vi "Actor Core.vi"(8 "error in":errorcluster, 11 "Menu View in":refnum<class "Menu View.lvclass">) -> (0 "error out":errorcluster, 3 "Actor out":refnum<class "Actor.lvclass">)   [LabVIEW 2020, in "Menu View.lvlib" / "Menu View.lvclass"]
doc: "(<B>Filename</B>: Actor Framework.lvlib:Actor.lvclass:Actor Core.vi)\n\nReceives messages to the actor, reacts to them, and initiates any error handling that may shut the actor down.\n\nDescendant classes may override this VI to append parallel tasks for the actor to complete while it handles messages. Overrides use the Call Parent Method node."
uses:
  Menu View.lvclass
  C:/Program Files/National Instruments/LabVIEW 2020/vi.lib/ActorFramework/Actor/Actor.lvclass
  <vilib>/ActorFramework/Actor/Actor.lvclass
  Menu View.lvclass/Menu View.ctl
  <vilib>/ActorFramework/Actor/Actor.lvclass/Actor.ctl
  <vilib>/ActorFramework/Message Enqueuer/Message Enqueuer.lvclass/Message Enqueuer.ctl
  Menu View Messages/Broadcast Menu Pressed Msg/Broadcast Menu Pressed Msg.lvclass/Broadcast Menu Pressed Msg.ctl
  Menu View Messages/Broadcast Tools Pressed Msg/Broadcast Tools Pressed Msg.lvclass/Broadcast Tools Pressed Msg.ctl
  Menu View Messages/Broadcast Help Pressed Msg/Broadcast Help Pressed Msg.lvclass/Broadcast Help Pressed Msg.ctl
  Menu View Messages/Broadcast Undo Pressed Msg/Broadcast Undo Pressed Msg.lvclass/Broadcast Undo Pressed Msg.ctl
  Menu View Messages/Broadcast Redo Pressed Msg/Broadcast Redo Pressed Msg.lvclass/Broadcast Redo Pressed Msg.ctl
  <vilib>/ActorFramework/Message Enqueuer/Init from Existing Queue.vi
  <vilib>/ActorFramework/Message Enqueuer/Enqueue.vi
  Menu View Messages/Broadcast Menu Pressed Msg/Broadcast Menu Pressed Msg.lvclass
  C:/Program Files/National Instruments/LabVIEW 2020/vi.lib/ActorFramework/Message/Message.lvclass
  Menu View Messages/Broadcast Tools Pressed Msg/Broadcast Tools Pressed Msg.lvclass
  Menu View Messages/Broadcast Help Pressed Msg/Broadcast Help Pressed Msg.lvclass
  Menu View Messages/Broadcast Undo Pressed Msg/Broadcast Undo Pressed Msg.lvclass
  Menu View Messages/Broadcast Redo Pressed Msg/Broadcast Redo Pressed Msg.lvclass
  <vilib>/ActorFramework/Message Priority Queue/Priority Enqueue.vi
  <vilib>/ActorFrameworkMVC/Abstract View/Abstract View/Abstract View.lvclass
  <vilib>/ActorFramework/Message Enqueuer/Message Enqueuer.lvclass
panel:
  in  "Tools Button":bool
  in  "Menu Button":bool
  in  "Help Button":bool
  in  "Disabled Redo Button":bool
  in  "Disabled Undo Button":bool
  in  "Undo Button":bool
  in  "Redo Button":bool
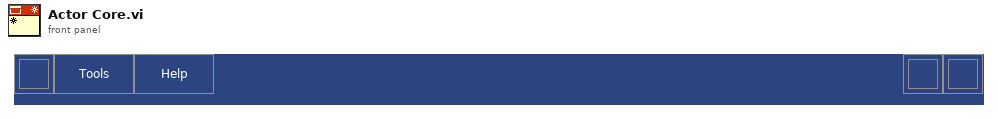
[diagram p1: front panel]
types:
  T1 = enum8{"Enabled", "Disabled", "Disabled and Grayed Out"}
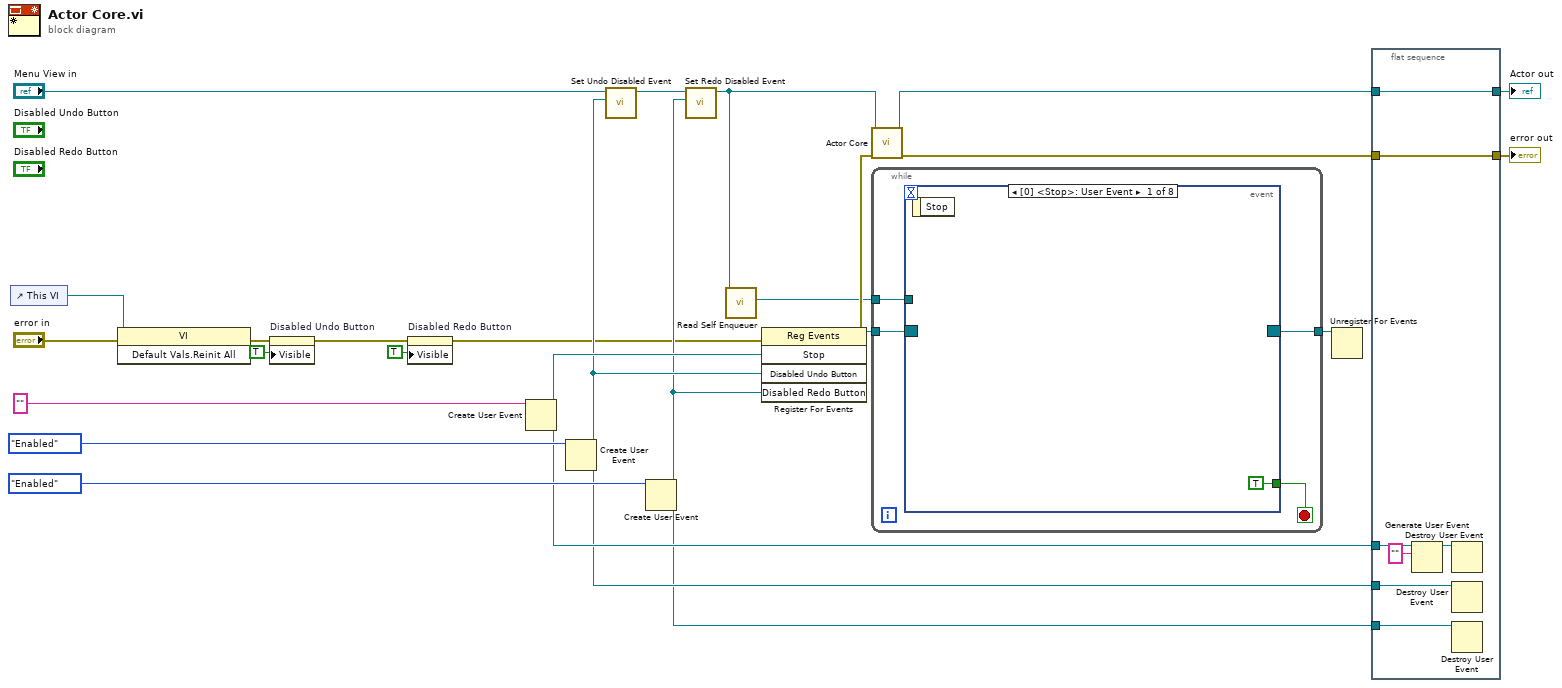
[diagram p0: block diagram]
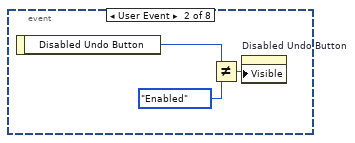
[diagram p2: hidden frame]
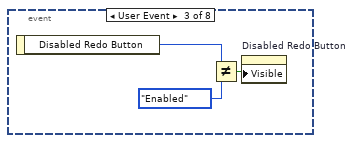
[diagram p3: hidden frame]
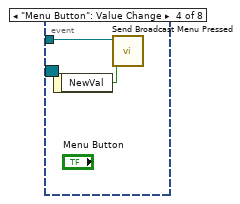
[diagram p4: hidden frame]
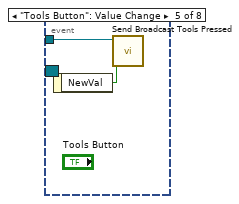
[diagram p5: hidden frame]
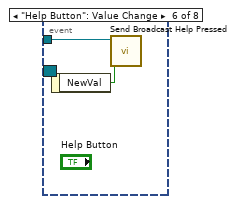
[diagram p6: hidden frame]
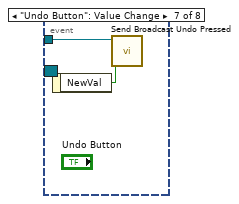
[diagram p7: hidden frame]
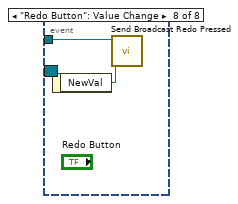
[diagram p8: hidden frame]
diagram:
  n1 = control-ref of="This VI"() -> (w6:refnum<vi>)
  n2 = invoke class="VI" method="Default Vals.Reinit All"(reference=w6, error in="error in") -> (error out=w5:errorcluster)  [unwired: 1 in, 2 out]
  n3 = property on="Disabled Undo Button" class="Bool"(error in=w5, "Visible"=TRUE) -> (error out=w4:errorcluster)  [unwired: 1 in, 1 out]
  n4 = property on="Disabled Redo Button" class="Bool"(error in=w4, "Visible"=TRUE) -> (error out=w3:errorcluster)  [unwired: 1 in, 1 out]
  n5 = Create User Event(user event datatype="" ("Stop")) -> (user event=w18:refnum<user-event>)  [unwired: 1 in, 1 out]
  n6 = Create User Event(user event datatype=T1."Enabled" ("Disabled Undo Button")) -> (user event=w12:refnum<user-event>)  [unwired: 1 in, 1 out]
  n7 = call "Set Undo Disabled Event.vi"("Undo Disabled Event"=w12, "Menu View in"="Menu View in") -> ("Menu View out"=w13:refnum<class "Menu View.lvclass">)  [unwired: 9 in]
  n8 = Create User Event(user event datatype=T1."Enabled" ("Disabled Redo Button")) -> (user event=w11:refnum<user-event>)  [unwired: 1 in, 1 out]
  n9 = call "Set Redo Disabled Event.vi"("Redo Disabled Event"=w11, "Menu View in"=w13) -> ("Menu View out"=w8:refnum<class "Menu View.lvclass">)  [unwired: 9 in]
  n10 = call <vilib>:"Read Self Enqueuer.vi"("Actor"=w8) -> ("Self Enqueuer"=w9:refnum<class "Message Enqueuer.lvclass">)  [unwired: 10 in]
  n11 = register-events(error in=w3, w18, w12, w11) -> (reference out=w23:refnum<event-registration>, error out=w10:errorcluster)  [unwired: 1 in]
  n12 = call-parent "Actor Core.vi"("error in"=w10, "Abstract View in"=w8) -> ("error out"=w14:errorcluster, "Actor out"=w17:refnum<class "Actor.lvclass">)  [unwired: 8 in]
  n13 = while {
    tunnel: w23 -> [w28]
    tunnel: [w27] -> w22
    tunnel: w9 -> [w25]
    stop <- w26 stop-if-true
    n14 = event shown="[0] <Stop>: User Event" {
      selector: w28 -> [_ _ _ _ _ _ _ _]
      dyn-events: [_ _ _ _ _ _ _ _] -> w27
      timeout: _ -> [_ _ _ _ _ _ _ _]
      tunnel: [TRUE _ _ _ _ _ _ _] -> w26
      tunnel: w25 -> [_ _ _ w37 w39 w40 w43 w45]
      event User Event {
        n15 = event-data() -> ()  [unwired: 1 in, 1 out]
      }
      event User Event {
        n16 = event-data() -> ("Disabled Undo Button"=w32:T1)  [unwired: 1 in]
        n17 = Not Equal?(x=w32, y=T1."Enabled") -> (x != y?=w30:bool)
        n18 = property on="Disabled Undo Button" class="Bool"("Visible"=w30) -> ()  [unwired: 2 in, 2 out]
      }
      event User Event {
        n19 = event-data() -> ("Disabled Redo Button"=w35:T1)  [unwired: 1 in]
        n20 = Not Equal?(x=w35, y=T1."Enabled") -> (x != y?=w33:bool)
        n21 = property on="Disabled Redo Button" class="Bool"("Visible"=w33) -> ()  [unwired: 2 in, 2 out]
      }
      event "Menu Button": Value Change {
        n22 = event-data() -> ("NewVal"=w36:bool)  [unwired: 1 in]
        n23 = call "Send Broadcast Menu Pressed.vi"("Menu Pressed"=w36, "Message Enqueuer"=w37) -> ()  [unwired: 8 in, 2 out]
      }
      event "Tools Button": Value Change {
        n24 = event-data() -> ("NewVal"=w38:bool)  [unwired: 1 in]
        n25 = call "Send Broadcast Tools Pressed.vi"("Tools Pressed"=w38, "Message Enqueuer"=w39) -> ()  [unwired: 8 in, 2 out]
      }
      event "Help Button": Value Change {
        n26 = event-data() -> ("NewVal"=w41:bool)  [unwired: 1 in]
        n27 = call "Send Broadcast Help Pressed.vi"("Help Pressed"=w41, "Message Enqueuer"=w40) -> ()  [unwired: 8 in, 2 out]
      }
      event "Undo Button": Value Change {
        n28 = event-data() -> ("NewVal"=w42:bool)  [unwired: 1 in]
        n29 = call "Send Broadcast Undo Pressed.vi"("Undo Pressed"=w42, "Message Enqueuer"=w43) -> ()  [unwired: 8 in, 2 out]
      }
      event "Redo Button": Value Change {
        n30 = event-data() -> ("NewVal"=w44:bool)  [unwired: 1 in]
        n31 = call "Send Broadcast Redo Pressed.vi"("Redo Pressed"=w44, "Message Enqueuer"=w45) -> ()  [unwired: 8 in, 2 out]
      }
    }
  }
  n32 = Unregister For Events(event registration refnum=w22) -> ()  [unwired: 1 in, 1 out]
  n33 = flat-sequence {
    tunnel: w18 -> [w51]
    tunnel: w12 -> [w49]
    tunnel: w11 -> [w48]
    tunnel: w17 -> [w47]
    tunnel: [w47] -> w16
    tunnel: [w46] -> w15
    tunnel: w14 -> [w46]
    frame #0 {
      n34 = Generate User Event(user event=w51, event data cluster="" ("event data")) -> (user event out=w52:refnum<user-event>)  [unwired: 2 in, 1 out]
      n35 = Destroy User Event(user event=w52) -> ()  [unwired: 1 in, 1 out]
      n36 = Destroy User Event(user event=w49) -> ()  [unwired: 1 in, 1 out]
      n37 = Destroy User Event(user event=w48) -> ()  [unwired: 1 in, 1 out]
    }
  }
  "error out" <- w15
  "Actor out" <- w16
